vi "IsItBlack.vi"(9 "End":i32, 10 "Start":i32, 11 "String in":refnum<vi>) -> (1 "Black?":bool, 3 "String out":refnum<vi>)   [LabVIEW 2019]
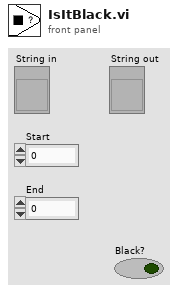
[diagram p1: front panel]
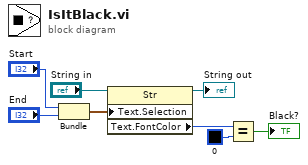
[diagram p0: block diagram]
diagram:
  n1 = Bundle("Start"="Start", "End"="End") -> (w4:cluster{"Start":i32, "End":i32})  [unwired: 1 in]
  n2 = property on="Property Node" class="Str"(reference="String in", "Text.Selection"=w4) -> (reference out=→"String out":refnum<vi>, "Text.FontColor"=w6:u32)  [unwired: 1 in, 1 out]
  n3 = Equal?(x=w6, y=u32 0 ("Color")) -> (x = y?=→"Black?":bool)
